vi "SP SP - click on ctrl.vi"(4 "subVI caller":refnum<vi>, 6 "subsubpanel":refnum<vi>, 7 "Control Label":string, 8 "error in (no error)":errorcluster, 9 "subpanel":refnum<vi>, 10 "subVI":refnum<vi>, 11 "VI with Focus":refnum<vi>) -> (0 "error out":errorcluster, 3 "return value":string)   [LabVIEW 2020, in "ui-testing.lvlib"]
uses:
  ui-testing.lvlib
  User32.dll
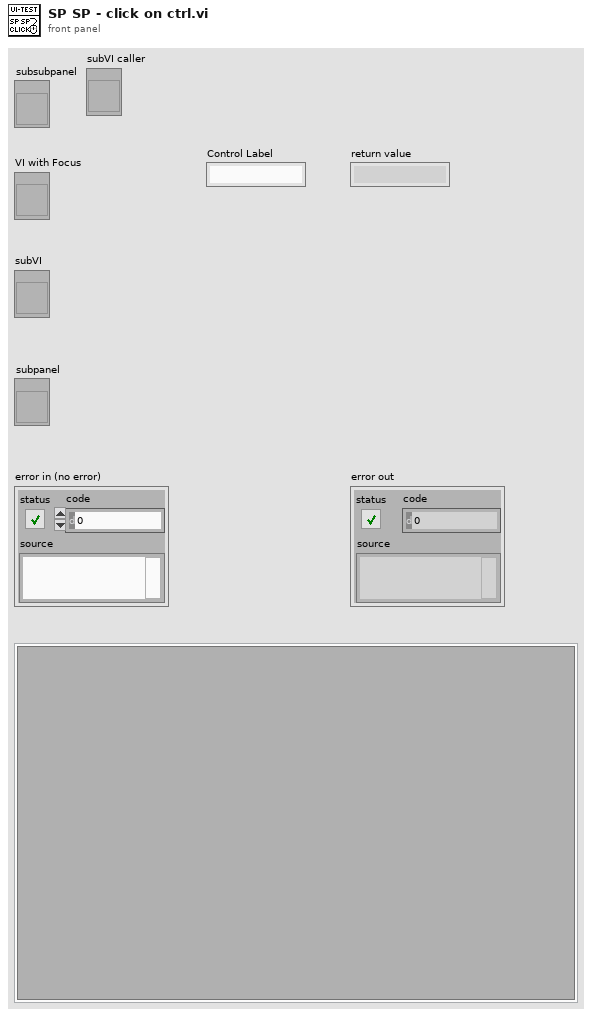
[diagram p1: front panel]
types:
  T1 = typedef "LVPositionTypeDef.ctl" = cluster{"Left":i32, "Top":i32}
  T2 = typedef "LVRectTypeDef.ctl" = cluster{"left":i16, "top":i16, "right":i16, "bottom":i16}
  T3 = typedef "LVPointTypeDef.ctl" = cluster{"Horizontal":i16, "Vertical":i16}
  T4 = typedef "LVBoundsTypeDef.ctl" = cluster{"Width":u32, "Height":u32}
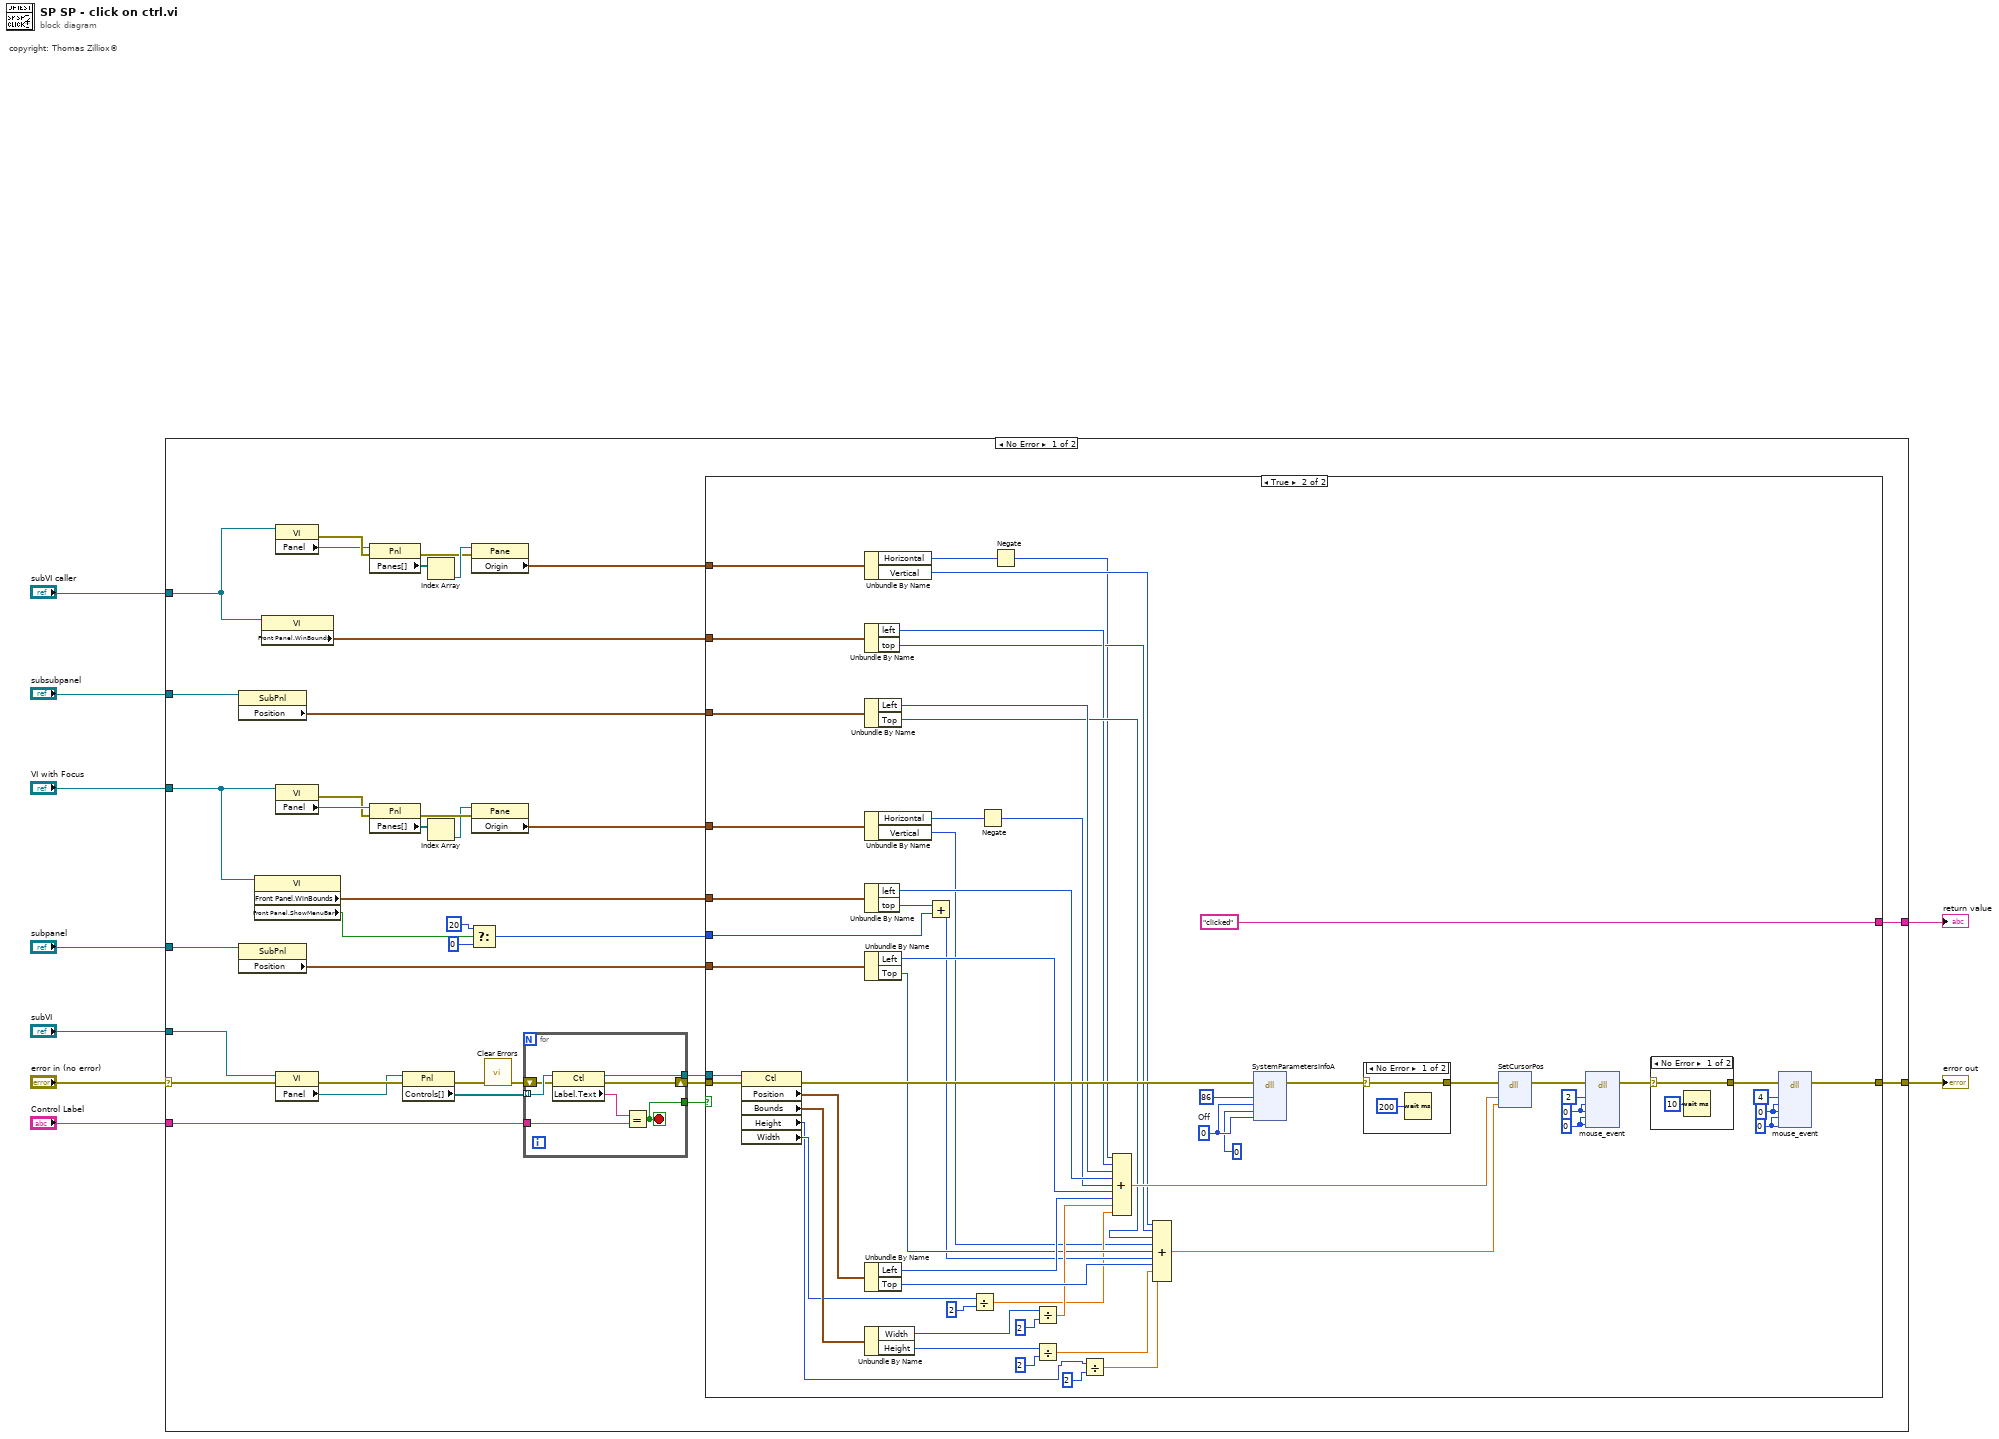
[diagram p0: block diagram]
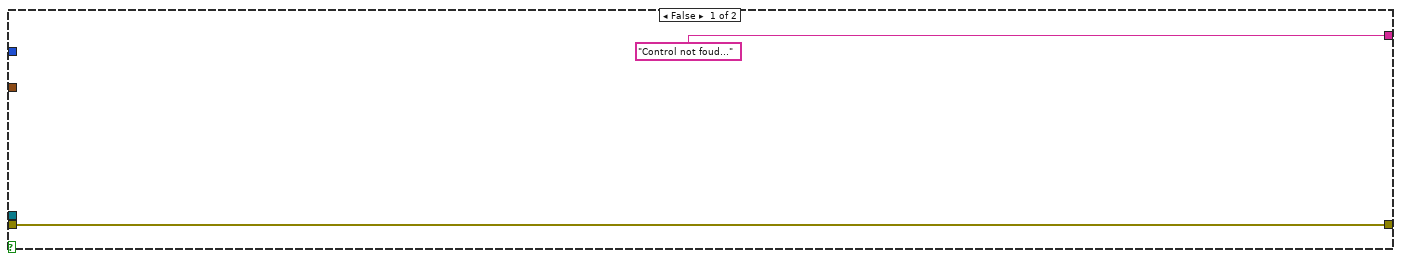
[diagram p2: hidden frame]
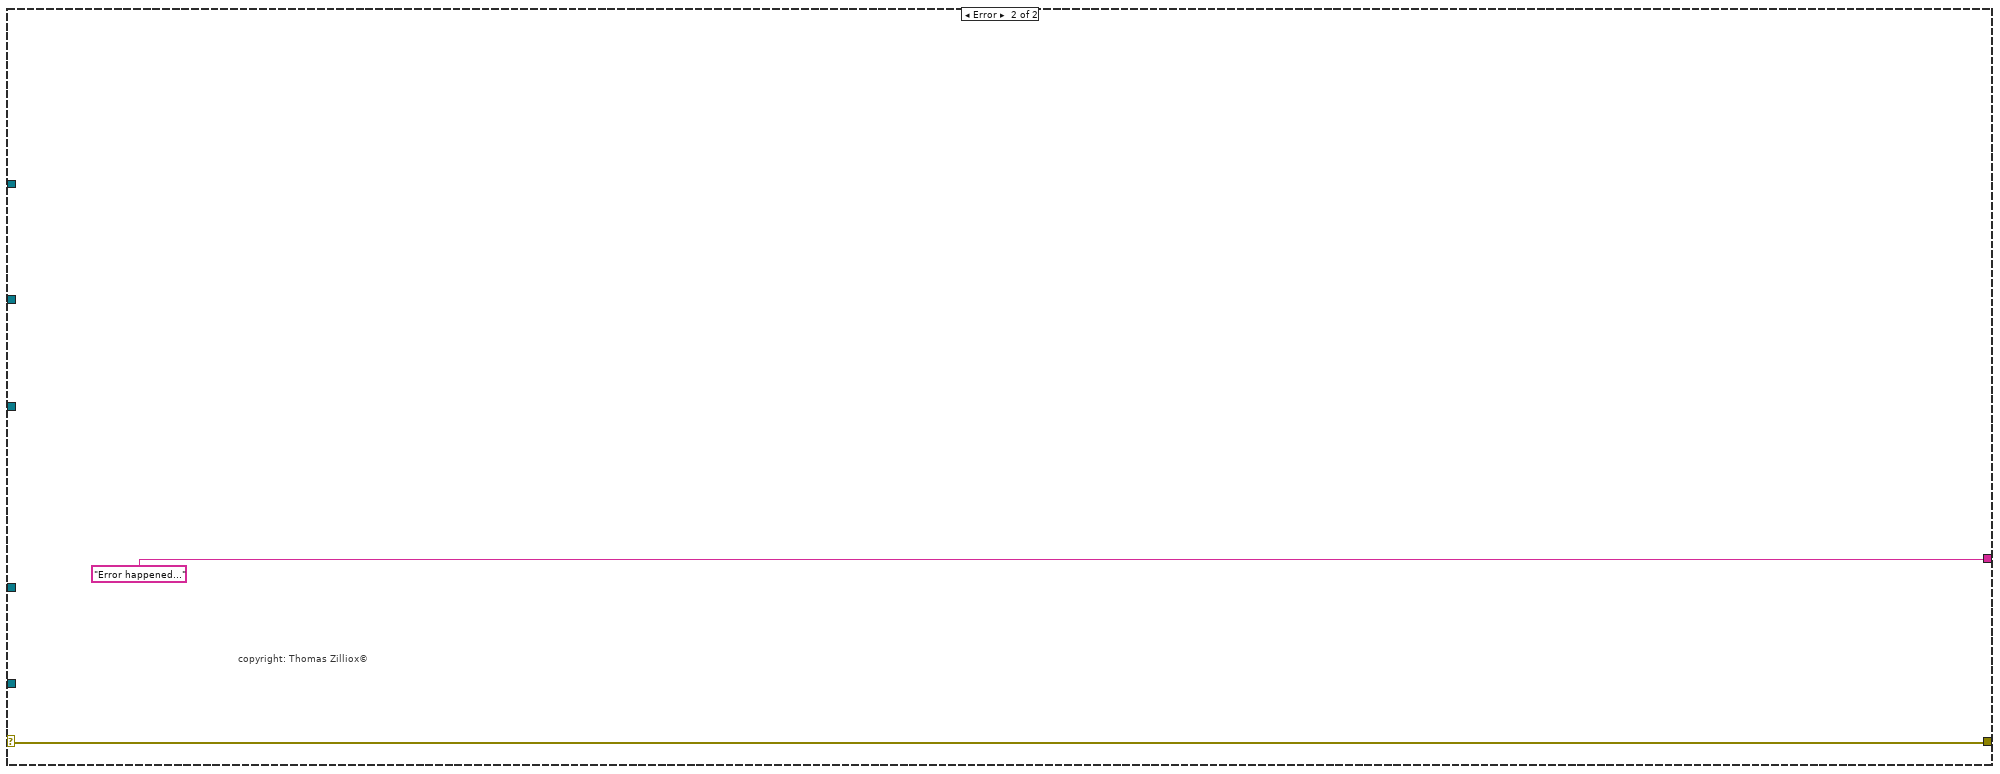
[diagram p5: hidden frame]
diagram:
  # "copyright: Thomas Zilliox©"
  n1 = case shown="No Error" "error in (no error)" {
    selector: "error in (no error)" -> [w28 w122]
    tunnel: [w29 w122] -> w8
    tunnel: "Control Label" -> [w32 _]
    tunnel: [w30 "Error happened..."] -> w6
    tunnel: "subVI" -> [w35 _]
    tunnel: "VI with Focus" -> [w34 _]
    tunnel: "subpanel" -> [w33 _]
    tunnel: "subsubpanel" -> [w23 _]
    tunnel: "subVI caller" -> [w16 _]
    frame No Error {
      n2 = property class="SubPnl"(reference=w23) -> ("Position"=w22:T1)  [unwired: 1 in, 2 out]
      n3 = property class="SubPnl"(reference=w33) -> ("Position"=w27:T1)  [unwired: 1 in, 2 out]
      n4 = property class="VI"(reference=w34) -> ("Front Panel.WinBounds"=w24:T2, "Front Panel.ShowMenuBar"=w13:bool)  [unwired: 1 in, 2 out]
      n5 = property class="VI"(reference=w16) -> ("Front Panel.WinBounds"=w15:T2)  [unwired: 1 in, 2 out]
      n6 = property class="VI"(reference=w16) -> (error out=w21:errorcluster, "Panel"=w20:refnum<vi>)  [unwired: 1 in, 1 out]
      n7 = property class="VI"(reference=w34) -> (error out=w26:errorcluster, "Panel"=w36:refnum<vi>)  [unwired: 1 in, 1 out]
      n8 = property class="VI"(reference=w35, error in=w28) -> (error out=w43:errorcluster, "Panel"=w40:refnum<vi>)  [unwired: 1 out]
      n9 = property class="Pnl"(reference=w20, error in=w21) -> (error out=w17:errorcluster, "Panes[]"=w18:refnum<vi>[])  [unwired: 1 out]
      n10 = property class="Pnl"(reference=w36, error in=w26) -> (error out=w39:errorcluster, "Panes[]"=w38:refnum<vi>[])  [unwired: 1 out]
      n11 = property class="Pnl"(reference=w40, error in=w43) -> (error out=w45:errorcluster, "Controls[]"=w46:refnum<vi>[])  [unwired: 1 out]
      n12 = Index Array(array=w18) -> (element=w19:refnum<vi>)  [unwired: 1 in]
      n13 = Index Array(array=w38) -> (element=w37:refnum<vi>)  [unwired: 1 in]
      n14 = Select(t=i16 20 ("top"), s=w13, f=i16 0) -> (s? t:f=w10:i16)
      n15 = property class="Pane"(reference=w19, error in=w17) -> ("Origin"=w14:T3)  [unwired: 2 out]
      n16 = property class="Pane"(reference=w37, error in=w39) -> ("Origin"=w25:T3)  [unwired: 2 out]
      n17 = call <vilib>:"Clear Errors.vi"("error in (no error)"=w45) -> ("error out"=w44:errorcluster)  [unwired: 5 in, 1 out]
      n18 = for {
        tunnel: w46 -> [w120] mode=indexing
        tunnel: w32 -> [w118]
        tunnel: [w117] -> w42
        shift-right: [w115] -> w41
        shift-left: w44 -> [w116]
        tunnel: [w114] -> w31
        stop <- w114 stop-if-true
        n19 = property class="Ctl"(reference=w120, error in=w116) -> (reference out=w117:refnum<vi>, error out=w115:errorcluster, "Label.Text"=w119:string)
        n20 = Equal?(x=w119, y=w118) -> (x = y?=w114:bool)
      }
      n21 = case shown="True" w31 {
        tunnel: w42 -> [_ w107]
        tunnel: w41 -> [w47 w106]
        tunnel: ["Control not foud..." ("VI Name") "clicked" ("VI Name")] -> w30
        tunnel: [w47 w73] -> w29
        tunnel: w27 -> [_ w88]
        tunnel: w25 -> [_ w86]
        tunnel: w24 -> [_ w63]
        tunnel: w22 -> [_ w72]
        tunnel: w15 -> [_ w69]
        tunnel: w14 -> [_ w64]
        tunnel: w10 -> [_ w60]
        frame False {
        }
        frame True {
          w79 = 0 ("dwExtraInfo")
          w80 = u32 0 ("dwExtraInfo")
          w78 = 0 ("dwExtraInfo")
          w77 = u32 0 ("dwExtraInfo")
          w105 = u32 0  # Off
          n22 = property class="Ctl"(reference=w107, error in=w106) -> (error out=w89:errorcluster, "Position"=w98:T1, "Bounds"=w97:T4, "Height"=w50:u32, "Width"=w56:u32)  [unwired: 1 out]
          n23 = Unbundle By Name(w64) -> ("Horizontal"=w68:i16, "Vertical"=w66:i16)
          n24 = Unbundle By Name(w69) -> ("left"=w67:i16, "top"=w65:i16)
          n25 = Unbundle By Name(w72) -> ("Left"=w71:i32, "Top"=w70:i32)
          n26 = Unbundle By Name(w86) -> ("Horizontal"=w85:i16, "Vertical"=w54:i16)
          n27 = Unbundle By Name(w63) -> ("left"=w84:i16, "top"=w83:i16)
          n28 = Unbundle By Name(w88) -> ("Left"=w87:i32, "Top"=w62:i32)
          n29 = Unbundle By Name(w98) -> ("Left"=w96:i32, "Top"=w94:i32)
          n30 = Unbundle By Name(w97) -> ("Width"=w95:u32, "Height"=w59:u32)
          n31 = Add(x=w83, y=w60) -> (x+y=w61:i16)
          n32 = Divide(x=w56, y=u32 2) -> (x/y=w55:dbl)
          n33 = Negate(x=w85) -> (-x=w52:i16)
          n34 = Negate(x=w68) -> (-x=w53:i16)
          n35 = Divide(x=w95, y=u32 2) -> (x/y=w93:dbl)
          n36 = Divide(x=w59, y=u32 2) -> (x/y=w58:dbl)
          n37 = Divide(x=w50, y=u32 2) -> (x/y=w49:dbl)
          n38 = Compound Arithmetic op=ADD(w53, w67, w71, w84, w52, w87, w96, w93, w55) -> (w100:dbl)
          n39 = Compound Arithmetic op=ADD(w66, w65, w70, w54, w62, w61, w94, w58, w49) -> (w99:dbl)
          n40 = dll-call lib="User32.dll" fn="SystemParametersInfoA" label="Terminate power-off mode"(error in=w89, "uiAction"=u32 86 ("SPI_GETPOWEROFFACTIVE"), "uiParam"=w105, "pvParam"=0, "fWinIni"=w105) -> (error out=w102:errorcluster)  [unwired: 7 in, 1 out]
          n41 = case shown="No Error" w102 {
            selector: w102 -> [w111 w113]
            tunnel: [w111 w113] -> w101
            frame No Error {
              n42 = Wait (ms)(milliseconds to wait=u32 200) -> ()  [unwired: 1 out]
            }
            frame Error {
            }
          }
          n43 = dll-call lib="User32.dll" fn="SetCursorPos" label="Move mouse"(error in=w101, "dx"=w100, "dy"=w99) -> (error out=w82:errorcluster)  [unwired: 5 in, 1 out]
          n44 = dll-call lib="User32.dll" fn="mouse_event" label="Click"(error in=w82, "dwFlags"=2, "dx"=w78, "dy"=w78, "dwData"=w77, "dwExtraInfo"=w77) -> (error out=w75:errorcluster)  [unwired: 8 in, 1 out]
          n45 = case shown="No Error" w75 {
            selector: w75 -> [w108 w110]
            tunnel: [w108 w110] -> w74
            frame No Error {
              n46 = Wait (ms)(milliseconds to wait=u32 10) -> ()  [unwired: 1 out]
            }
            frame Error {
            }
          }
          n47 = dll-call lib="User32.dll" fn="mouse_event" label="Release"(error in=w74, "dwFlags"=4, "dx"=w79, "dy"=w79, "dwData"=w80, "dwExtraInfo"=w80) -> (error out=w73:errorcluster)  [unwired: 8 in, 1 out]
        }
      }
    }
    frame Error {
      # "copyright: Thomas Zilliox©"
    }
  }
  "error out" <- w8
  "return value" <- w6
